vi "Stress test Hard drive1.vi"() -> ()   [LabVIEW 2022 SP3]
panel:
  out "Time per file Seconds":dbl(graph)
  out "Hours Running":dbl
  out "Number of loops":i32
  out "Filename":string
  out "File number":i32
  in  "stop":bool
  in  "Please select folder":path
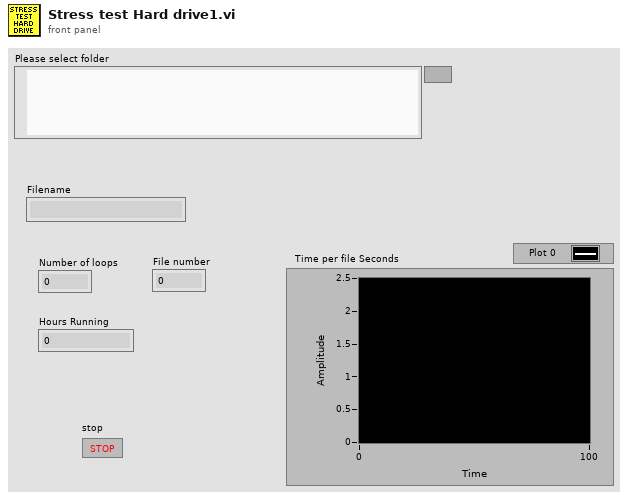
[diagram p1: front panel]
types:
  T1 = enum16{"open", "replace", "create", "open or create", "replace or create", "replace or create with confirmation"}
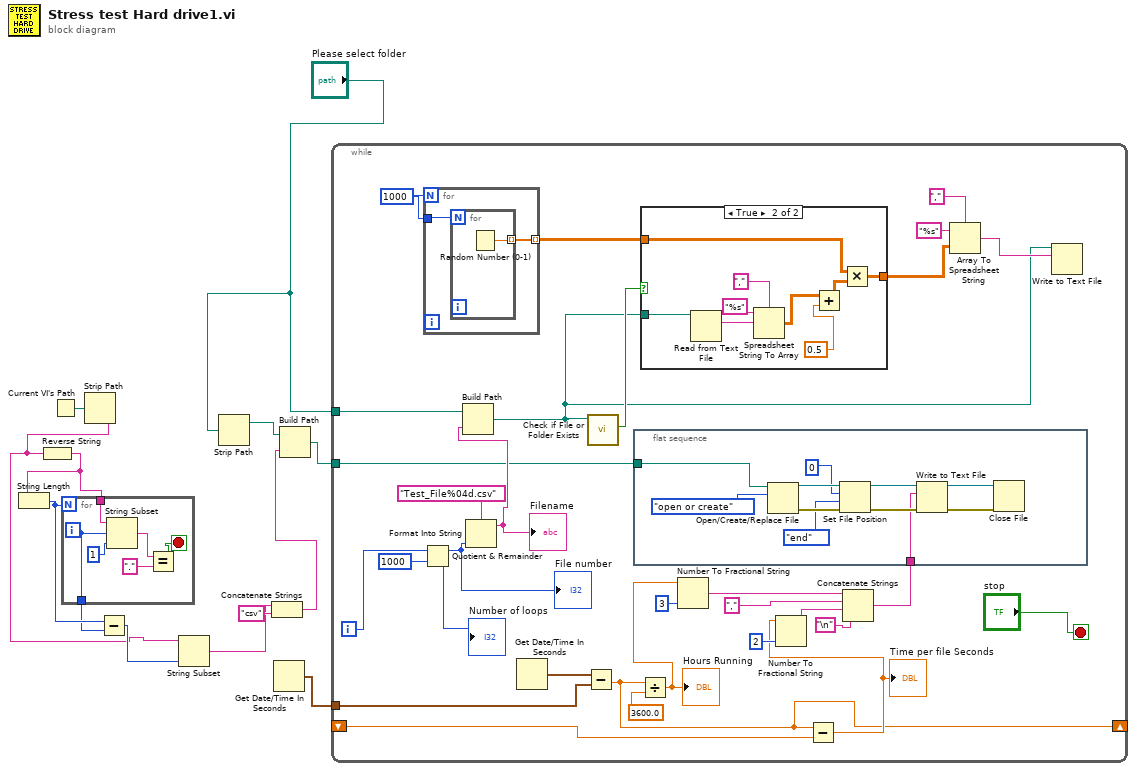
[diagram p0: block diagram]
diagram:
  n1 = Current VI's Path() -> (path=w12:path)
  n2 = Strip Path(path=w12) -> (name=w2:string)  [unwired: 1 out]
  n3 = Reverse String(1:w2) -> (0:w6:string)
  n4 = String Length(string=w6) -> (length=w5:i32)
  n5 = for {
    N: w5 -> [_]
    tunnel: w6 -> [w18]
    tunnel: [w14] -> w4
    i -> [w14]
    stop <- w15 stop-if-true
    n6 = String Subset(string=w18, offset (0)=w14, length (rest)=1 ("length (rest)")) -> (substring=w17:string)
    n7 = Equal?(x=w17, y=".") -> (x = y?=w15:bool)
  }
  n8 = Subtract(x=w5, y=w4) -> (x-y=w3:i32)
  n9 = String Subset(string=w2, length (rest)=w3) -> (substring=w1:string)  [unwired: 1 in]
  n10 = Strip Path(path="Please select folder") -> (stripped path=w10:path)  [unwired: 1 out]
  n11 = Concatenate Strings(w1, "csv" ("string")) -> (w7:string)
  n12 = Get Date/Time In Seconds() -> (seconds since 1Jan1904=w13:timestamp)
  n13 = Build Path(base path=w10, name or relative path=w7) -> (appended path=w9:path)
  n14 = while {
    tunnel: "Please select folder" -> [w31]
    tunnel: w13 -> [w34]
    shift-right: [w20] -> _
    shift-left: _ -> [w32]
    tunnel: w9 -> [w30]
    i -> [w48]
    stop <- "stop" stop-if-true
    w50 = 1000
    n15 = Quotient & Remainder(x=w48, y=1000) -> (x-y*floor(x/y)=w46:i32, floor(x/y)=→"Number of loops":i32)
    "File number" <- w46
    n16 = for {
      N: w50 -> [_]
      tunnel: [w73] -> w42 mode=indexing
      tunnel: w50 -> [w72]
      n17 = for {
        N: w72 -> [_]
        tunnel: [w74] -> w73 mode=indexing
        n18 = Random Number (0-1)() -> (number: 0 to 1=w74:dbl)
      }
    }
    n19 = Format Into String(format string="Test_File%04d.csv", w46) -> (resulting string=w44:string)  [unwired: 2 in, 1 out]
    "Filename" <- w44
    n20 = Build Path(base path=w31, name or relative path=w44) -> (appended path=w37:path)
    n21 = Get Date/Time In Seconds() -> (seconds since 1Jan1904=w35:timestamp)
    n22 = Subtract(x=w35, y=w34) -> (x-y=w20:dbl)
    n23 = call <vilib>:"Check if File or Folder Exists.vi"("path"=w37) -> ("file or folder exists?"=w43:bool)  [unwired: 1 in, 9 out]
    n24 = flat-sequence {
      tunnel: w30 -> [w61]
      tunnel: w22 -> [w51]
      frame #0 {
        n25 = Open/Create/Replace File(file path (use dialog)=w61, operation (0:open)=T1."open or create") -> (refnum out=w59:refnum<file>, error out=w56:errorcluster)  [unwired: 4 in, 1 out]
        n26 = Set File Position(offset (in bytes) (0)=i64 0, refnum=w59, from (0:start)=enum16{"start", "end", "current"}."end", error in=w56) -> (refnum out=w58:refnum<file>, error out=w57:errorcluster)
        n27 = Write to Text File(file (use dialog)=w58, text=w51, error in=w57) -> (refnum out=w53:refnum<file>, error out=w52:errorcluster)  [unwired: 1 in, 1 out]
        n28 = Close File(refnum=w53, error in=w52) -> ()  [unwired: 2 out]
      }
    }
    n29 = Divide(x=w20, y=3600.0) -> (x/y=w21:dbl)
    "Hours Running" <- w21
    n30 = case shown="True" w43 {
      tunnel: w37 -> [_ w71]
      tunnel: w42 -> [w62 w64]
      tunnel: [w62 w63] -> w38
      frame False {
      }
      frame True {
        n31 = Read from Text File(file (use dialog)=w71) -> (text=w70:string)  [unwired: 3 in, 3 out]
        n32 = Spreadsheet String To Array(delimiter (Tab)=",", format string="%s", spreadsheet string=w70) -> (array=w66:dbl[][])  [unwired: 1 in]
        n33 = Add(x=w66, y=0.5) -> (x+y=w65:dbl[][])
        n34 = Multiply(x=w64, y=w65) -> (x*y=w63:dbl[][])
      }
    }
    n35 = Number To Fractional String(number=w21, precision (6)=i16 3) -> (F-format string=w28:string)  [unwired: 2 in]
    n36 = Subtract(x=w20, y=w32) -> (x-y=w25:dbl)
    "Time per file Seconds" <- w25
    n37 = Number To Fractional String(number=w25, precision (6)=i16 2) -> (F-format string=w24:string)  [unwired: 2 in]
    n38 = Concatenate Strings(w28, "," ("string"), w24, "\n") -> (w22:string)
    n39 = Array To Spreadsheet String(delimiter (Tab)=",", array=w38, 3:"%s" ("format string")) -> (spreadsheet string=w41:string)
    n40 = Write to Text File(file (use dialog)=w37, text=w41) -> ()  [unwired: 2 in, 3 out]
  }
